vi "DatReadColumn.vi"(6 "error in (no error)":errorcluster, 8 "Names":string[](array[string])=["par1", "par2"], 9 "tracename":string="F:\\2017 10 06\\current vi's\\Data\\data_025.tdms: 2") -> (0 "error out":errorcluster, 1 "Values out":dbl[][](array[numeric])=[[1.0, 2.0]], 3 "tracename out":string)   [LabVIEW 2018]
uses:
  <vilib>/Utility/file.llb/Read From Spreadsheet File (string).vi
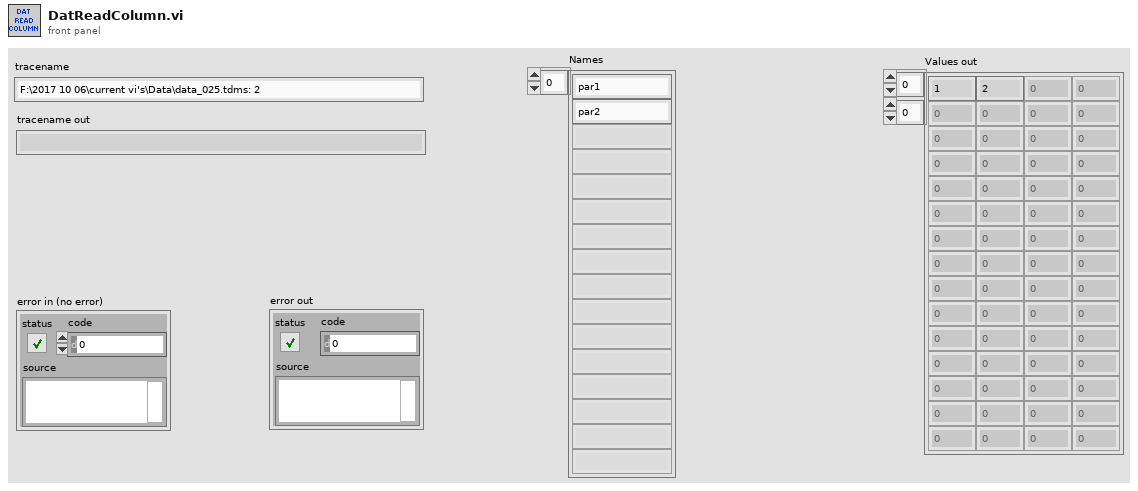
[diagram p1: front panel]
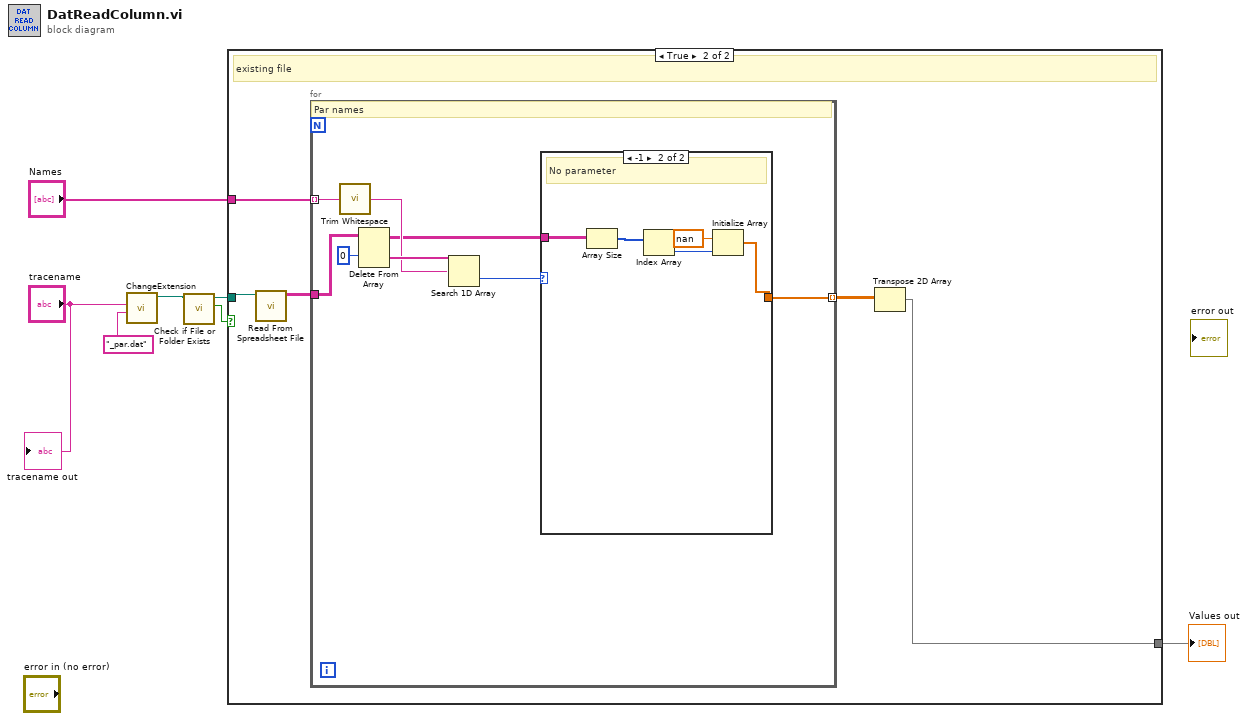
[diagram p0: block diagram]
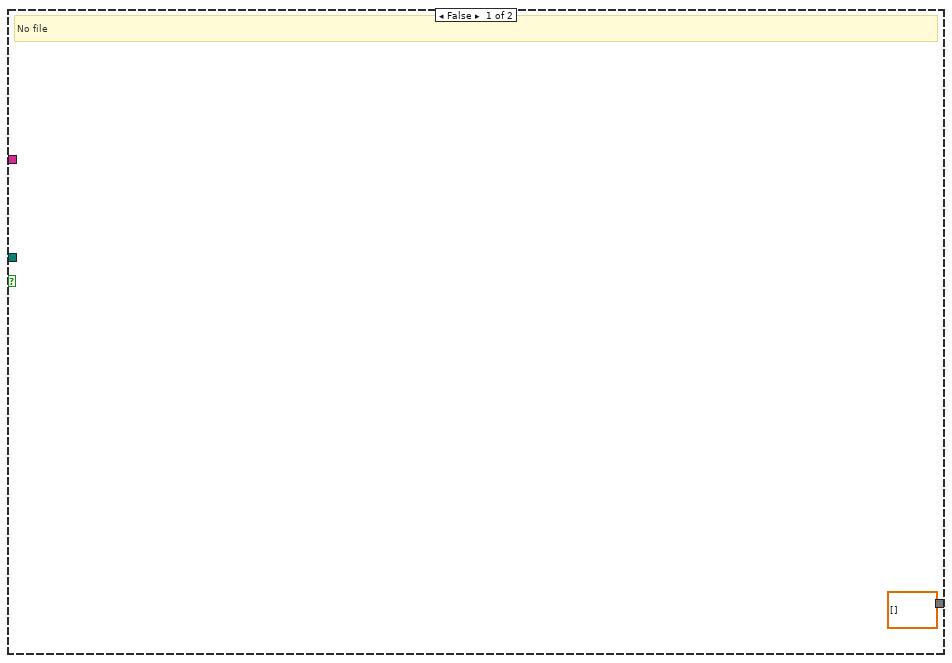
[diagram p2: hidden frame]
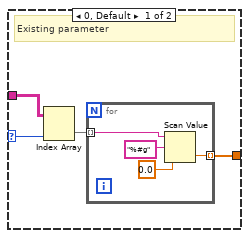
[diagram p3: hidden frame]
diagram:
  n1 = call "ChangeExtension.vi"("extension"="_par.dat", "file in"="tracename") -> ("Path out"=w4:path)  [unwired: 3 in, 4 out]
  n2 = call <vilib>:"Check if File or Folder Exists.vi"("path"=w4) -> ("file or folder exists?"=w2:bool, "dup path"=w3:path)  [unwired: 8 in, 1 out]
  n3 = case shown="True" w2 {
    tunnel: "Names" -> [_ w13]
    tunnel: w3 -> [_ w12]
    tunnel: [dbl[][] [] w9] -> w1
    frame False {
      # "No file"
    }
    frame True {
      # "existing file"
      n4 = call-poly <vilib>:"Read From Spreadsheet File.vi"("file path (dialog if empty)"=w12) -> ("all rows"=w11:string[][])  [unwired: 6 in, 4 out]
      n5 = for {
        tunnel: w13 -> [w21] mode=indexing
        tunnel: w11 -> [w16]
        tunnel: [w18] -> w10 mode=indexing
        # "Par names"
        n6 = call <vilib>:"Trim Whitespace.vi"("string"=w21) -> ("trimmed string"=w15:string)  [unwired: 1 in]
        n7 = Delete From Array(array=w16, index (row)=0) -> (deleted portion=w19:string[], array with subset deleted=w14:string[][])  [unwired: 2 in]
        n8 = Search 1D Array(1D array=w19, element=w15) -> (index of element=w17:i32)  [unwired: 1 in]
        n9 = case shown="-1" w17 {
          selector: w17 -> [w25 _]
          tunnel: [w22 w30] -> w18
          tunnel: w14 -> [w24 w34]
          frame 0, Default {
            # "Existing parameter"
            n10 = Index Array(array=w24, index (col)=w25) -> (element=w23:string[])  [unwired: 1 in]
            n11 = for {
              tunnel: w23 -> [w28] mode=indexing
              tunnel: [w27] -> w22 mode=indexing
              n12 = Scan Value(string=w28, format string="%#g", default (0 dbl)=0.0) -> (value=w27:dbl)  [unwired: 1 out]
            }
          }
          frame -1 {
            # "No parameter"
            n13 = Array Size(array=w34) -> (size(s)=w33:i32[])
            n14 = Index Array(array=w33) -> (element=w32:i32)  [unwired: 1 in]
            n15 = Initialize Array(nan ("element"), w32) -> (w30:dbl[])
          }
        }
      }
      n16 = Transpose 2D Array(2D array=w10) -> (transposed array=w9:dbl[][])
    }
  }
  "Values out" <- w1
  "tracename out" <- "tracename"
